vi "5.1.vi"() -> ()   [LabVIEW 2023]
panel:
  in  "stop":bool
  in  "DO Lines":bool[](array[boolean])=[TRUE, FALSE, FALSE, FALSE, FALSE, FALSE, FALSE, FALSE]
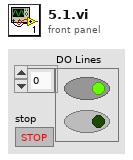
[diagram p1: front panel]
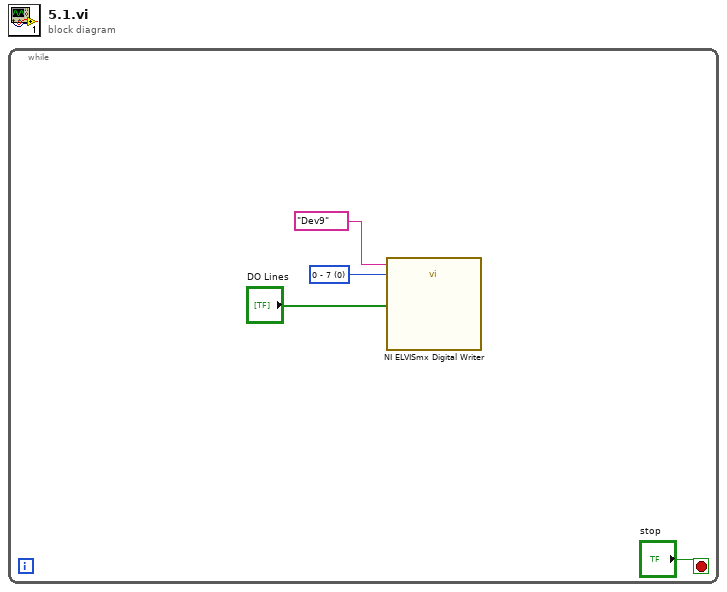
[diagram p0: block diagram]
diagram:
  n1 = while {
    stop <- "stop" stop-if-true
    w1 = u16 0 items=["0 - 7", "8 - 15", "16 - 23"] ("Lines to Write")
    n2 = call "NI ELVISmx Digital Writer"("Device Name"=tag "Dev9", "Lines to Write"=w1, "DO Lines"="DO Lines") -> ()  [unwired: 16 in, 1 out]
  }
